vi "Wavelet Order Selection.vi"() -> ()   [LabVIEW 2023]
doc: "This example shows how to select the order of wavelets. If the order of a wavelet is high enough, the detail coefficients are closer to zero. This example uses a polynomial as the signal under analysis. When the wavelet order is high enough, the polynomial can be approximated perfectly by the approximation coefficients if the border distortion is neglected.\n\n<b>Instructions:</b>\n1) Run this VI.\n2) Change the <b>Wavelet</b> type. The numbers following the <b>Wavelet</b> indicate the order of the wavelet.\n3) Observe the <b>Approximation and Detail Coefficients</b>.\n4) Notice that when the order of the wavelet is higher than the polynomial order, the detail coefficients are closer to zero."
uses:
  <vilib>/Analysis/1siggen.llb/Ramp Pattern by Samples.vi
  <vilib>/Analysis/polynomials.llb/1D Polynomial Evaluation (DBL).vi
  <vilib>/addons/Wavelet Analysis/filter banks.llb/WA 1D Analysis Filter Bank (Array).vi
  <vilib>/addons/_Advanced Signal Processing/NI_AdvSigProcWA.lvlib
  <vilib>/Analysis/NI_AALPro.lvlib
  <vilib>/Analysis/NI_AALBase.lvlib
panel:
  in  "stop":bool
  out "Perfect Approximation?":bool
  out "Approximation and Detail Coefficients":dbl[][](graph)
  out "Part of Detail Coefficients (64-192)":dbl[](graph)
  in  "Wavelet":u16(ring) items=["db02"=0, "db03"=1, "db04"=2, "db05"=3, "db06"=4, "db07"=5, "db08"=6, "db09"=7, "db10"=8, "db11"=9, "db12"=10, "db13"=11, "db14"=12, "Haar"=13, "bior1_3"=14, "bior1_5"=15, "bior2_2"=16, "bior2_4"=17, "bior2_6"=18, "bior2_8"=19, "bior3_1"=20, "bior3_3"=21, "bior3_5"=22, "bior3_7"=23, "bior3_9"=24, "bior4_4 (FBI)"=25, "bior5_5"=38, "bior6_8"=39, "coif1"=26, "coif2"=27, "coif3"=28, "coif4"=29, "coif5"=30, "sym2"=31, "sym3"=32, "sym4"=33, "sym5"=34, "sym6"=35, "sym7"=36, "sym8"=37]
  out "Polynomial":dbl[](graph)
  in  "P(x)":dbl[](array[numeric])=[0.0, 0.2, 1.0, -0.1]
  # "Overview: Shows how to select the order of wavelets. If the order of a wavelet is high enough, the detail coefficients are closer to zero. \nRequirements: LabVIEW Full Development System, Advanced Signal Processing Toolkit\nInstructions: \n1. Run this VI.\n2. Change the Wavelet type. The numbers following the Wavelet indicate the order of the wavelet.\n3. Observe the Approximation and Detail Coefficients.\n4. Notice that when the order of the wavelet is higher than the polynomial order, the detail coefficients are closer to zero.\n5. Click Stop to stop the VI."
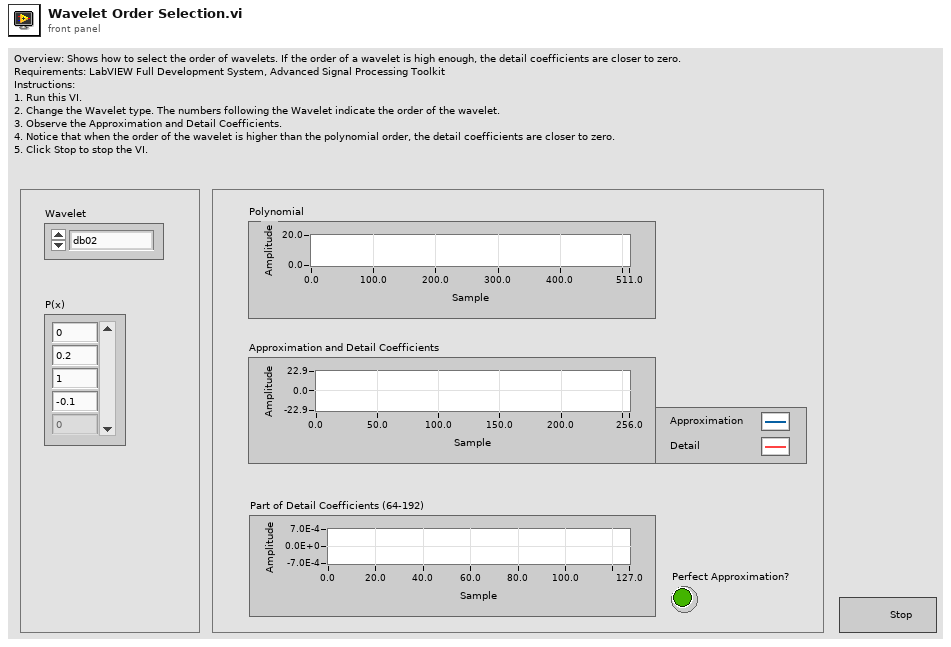
[diagram p1: front panel]
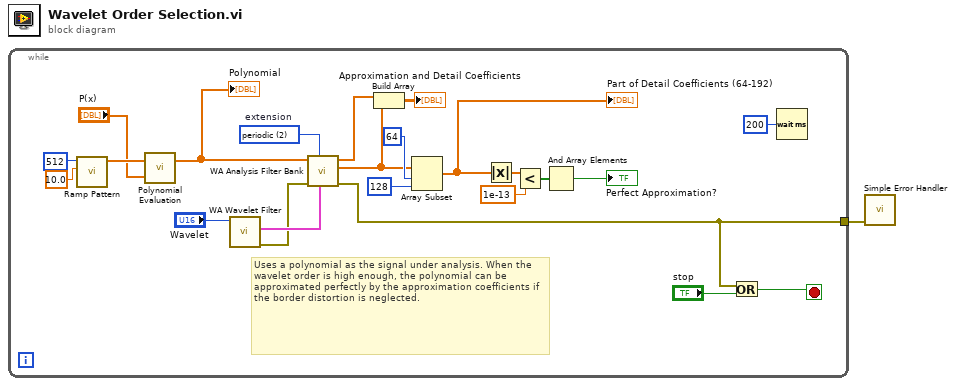
[diagram p0: block diagram]
diagram:
  n1 = while {
    tunnel: [w3] -> w1
    stop <- w5 stop-if-true
    w20 = u16 2 items=["zero padding", "symmetric", "periodic", "spline"]  # extension
    # "Uses a polynomial as the signal under analysis. When the wavelet order is high enough, the polynomial can be approximated perfectly by the approximation coefficients if the border distortion is neglected."
    n2 = call-poly <vilib>:"Ramp Pattern.vi"("end"=10.0, "samples"=512) -> ("Ramp Pattern"=w24:dbl[])  [unwired: 8 in, 1 out]
    n3 = call-poly <vilib>:"Polynomial Evaluation.vi"("P(x)"="P(x)", "A"=w24) -> ("P(A)"=w21:dbl[])  [unwired: 1 out]
    "Polynomial" <- w21
    n4 = call <vilib>:"WA Wavelet Filter.vi"("wavelet"="Wavelet") -> ("error out"=w2:errorcluster, "analysis filters"=w17:cluster{"lowpass":dbl[], "highpass":dbl[]})  [unwired: 3 in, 6 out]
    n5 = call-poly <vilib>:"WA Analysis Filter Bank.vi"("analysis filters"=w17, "extension"=w20, "error in (no error)"=w2, "signal"=w21) -> ("error out"=w3:errorcluster, "detail coef"=w7:dbl[], "approx coef"=w8:dbl[])  [unwired: 5 out]
    n6 = Build Array(w8, w7) -> (→"Approximation and Detail Coefficients":dbl[][])
    n7 = Array Subset(array=w7, index=64, length=128) -> (w13:dbl[])
    "Part of Detail Coefficients (64-192)" <- w13
    n8 = Absolute Value(x=w13) -> (abs(x)=w12:dbl[])
    n9 = Less?(x=w12, y=1e-13) -> (x < y?=w10:bool[])
    n10 = And Array Elements(Boolean array=w10) -> (logical AND=→"Perfect Approximation?":bool)
    n11 = Or(x=w3, y="stop") -> (x .or. y?=w5:bool)
    n12 = Wait (ms)(milliseconds to wait=u32 200 ("millisecond multiple")) -> ()  [unwired: 1 out]
  }
  n13 = call <vilib>:"Simple Error Handler.vi"("error in (no error)"=w1) -> ()  [unwired: 1 in, 8 out]
